vi "RobotProfileParser.vi"(0 "Selected Robot":i32) -> ()   [LabVIEW 2019]
doc: "Uses robot profile information to determine which sensors should be bypassed"
uses:
  robotprofile.vi
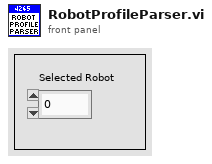
[diagram p1: front panel]
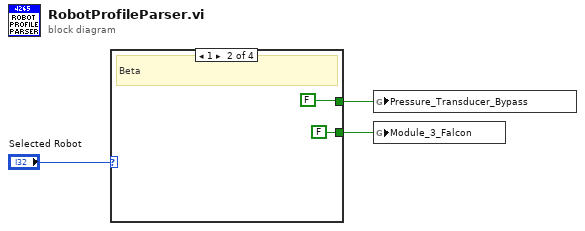
[diagram p0: block diagram]
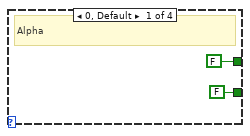
[diagram p2: hidden frame]
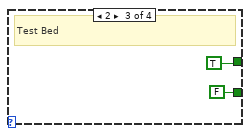
[diagram p3: hidden frame]
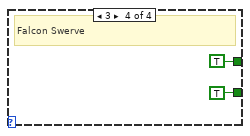
[diagram p4: hidden frame]
diagram:
  n1 = case shown="1" "Selected Robot" {
    tunnel: [FALSE ("Pressure_Transducer_Bypass") FALSE ("Pressure_Transducer_Bypass") TRUE ("Pressure_Transducer_Bypass") TRUE ("Pressure_Transducer_Bypass")] -> w2
    tunnel: [FALSE ("Pressure_Transducer_Bypass") FALSE ("Pressure_Transducer_Bypass") FALSE ("Pressure_Transducer_Bypass") TRUE ("Pressure_Transducer_Bypass")] -> w1
    frame 0, Default {
      # "Alpha"
    }
    frame 1 {
      # "Beta"
    }
    frame 2 {
      # "Test Bed"
    }
    frame 3 {
      # "Falcon Swerve"
    }
  }
  n2 = global write "robotprofile.vi" "Pressure_Transducer_Bypass"(w2) -> ()
  n3 = global write "robotprofile.vi" "Module_3_Falcon"(w1) -> ()
